vi "rtin_ControlMoveGPIO.vi"(7 "Set":bool, 8 "error in":errorcluster, 9 "Enable":bool, 10 "axis in":u8, 11 "connection ID":refnum<k5>) -> (0 "error out":errorcluster, 1 "Enable out":bool, 2 "axis out":i32, 3 "connection ID":refnum<k5>)   [LabVIEW 2015, in "AMC_VIs.lvlib"]
doc: "This function retrieves or sets the status for real time input on the selected axis in closed-loop mode."
uses:
  AMC_VIs.lvlib
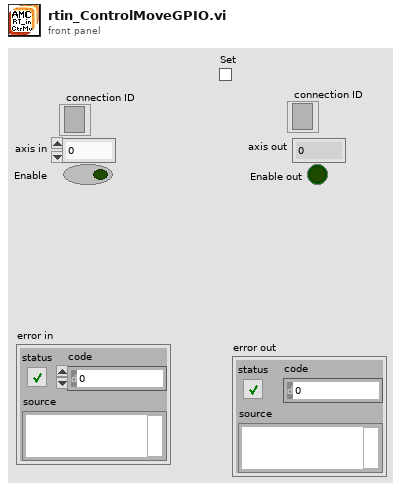
[diagram p1: front panel]
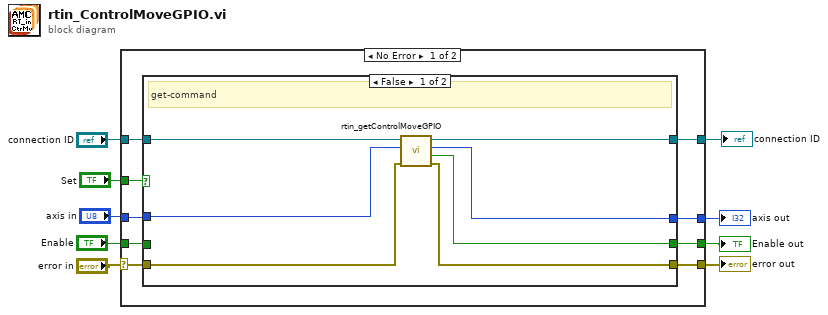
[diagram p0: block diagram]
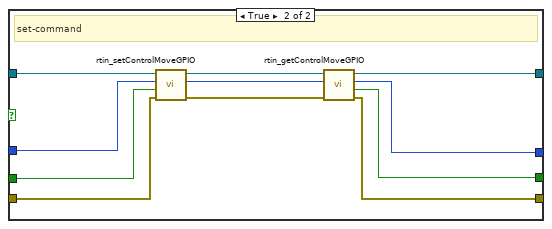
[diagram p2: hidden frame]
diagram:
  n1 = case shown="No Error" "error in" {
    selector: "error in" -> [w14 w40]
    tunnel: "axis in" -> [w18 w37]
    tunnel: [w11 w40] -> w8
    tunnel: "Enable" -> [w16 w38]
    tunnel: [w13 w38] -> w3
    tunnel: "Set" -> [w15 _]
    tunnel: [w12 w39] -> w6
    tunnel: "connection ID" -> [w17 w39]
    tunnel: [w10 w37] -> w1
    frame No Error {
      n2 = case shown="False" w15 {
        tunnel: w17 -> [w25 w33]
        tunnel: w18 -> [w21 w28]
        tunnel: w16 -> [_ w29]
        tunnel: w14 -> [w23 w31]
        tunnel: [w19 w27] -> w13
        tunnel: [w24 w32] -> w12
        tunnel: [w22 w30] -> w11
        tunnel: [w20 w26] -> w10
        frame False {
          # "get-command"
          n3 = call "rtin_getControlMoveGPIO.vi"("error in"=w23, "axis"=w21, "connection ID"=w25) -> ("error out"=w22:errorcluster, "enable"=w19:bool, "axis_out"=w20:i32, "connection ID"=w24:refnum<k5>)  [unwired: 5 in]
        }
        frame True {
          # "set-command"
          n4 = call "rtin_setControlMoveGPIO.vi"("error in"=w31, "enable"=w29, "axis"=w28, "connection ID"=w33) -> ("error out"=w34:errorcluster, "axis_out"=w36:i32, "connection ID"=w35:refnum<k5>)  [unwired: 5 in]
          n5 = call "rtin_getControlMoveGPIO.vi"("error in"=w34, "axis"=w36, "connection ID"=w35) -> ("error out"=w30:errorcluster, "enable"=w27:bool, "axis_out"=w26:i32, "connection ID"=w32:refnum<k5>)  [unwired: 5 in]
        }
      }
    }
    frame Error {
    }
  }
  "error out" <- w8
  "axis out" <- w1
  "Enable out" <- w3
  "connection ID" <- w6
